vi "ZLIB Extract Stream__ogtk.vi"(4 "password (none)":string, 6 "error in (no error)":errorcluster, 7 "internal name":string, 9 "unzip Refnum":T1) -> (0 "error out":errorcluster, 2 "byte stream":string, 3 "unzip Refnum out":T1)   [LabVIEW 2014]
doc: "Extracts a file in an unzip session to a target path."
uses:
  ZLIB Unzip Handle__ogtk.ctl
panel:
  out "read only":bool
  # "Please visit http://www.OpenG.org to learn about the\nOpen Source LabVIEW software movement.\n\nNOTICE -- YOU MUST LEAVE THIS NOTICE IN PLACE.  PER THE TERMS OF THE LICENSE BELOW, YOU MAY SUBLICENSE THIS SOFTWARE \nIN ANY WAY THAT DOES NOT CONFLICT WITH THIS LICENSE.\n\n### BSD License (http://www.opensource.org/licenses/bsd-license.php) Begin ###\n \nCopyright (C) 2002-2007 Rolf Kalbermatter rolf.kalbermatter@citeng.com\nCopyright (C) 2002 Jim Kring jim@jimkring.com\n\nAll rights reserved.\n\nRedistribution and use in source and binary forms, with or without modification, are permitted provided that the following conditions are met:\n\n    * Redistributions of source code must retain the above copyright notice, this list of conditions and the following disclaimer.\n    * Redistributions in binary form must reproduce the above copyright notice, this list of conditions and the following disclaimer in the \n       documentation and/or other materials provided with the distribution.\n    * Neither the name of SciWare, James Kring, Inc., nor the names of its contributors may be used to endorse or promote products derived \n       from this software without specific prior written permission.\n\nTHIS SOFTWARE IS PROVIDED BY THE COPYRIGHT HOLDERS AND CONTRIBUTORS \"AS IS\" AND ANY EXPRESS OR IMPLIED WARRANTIES, \nINCLUDING, BUT NOT LIMITED TO, THE IMPLIED WARRANTIES OF MERCHANTABILITY AND FITNESS FOR A PARTICULAR PURPOSE ARE \nDISCLAIMED. IN NO EVENT SHALL THE COPYRIGHT OWNER OR CONTRIBUTORS BE LIABLE FOR ANY DIRECT, INDIRECT, INCIDENTAL,\n SPECIAL, EXEMPLARY, OR CONSEQUENTIAL DAMAGES (INCLUDING, BUT NOT LIMITED TO, PROCUREMENT OF SUBSTITUTE GOODS OR \nSERVICES; LOSS OF USE, DATA, OR PROFITS; OR BUSINESS INTERRUPTION) HOWEVER CAUSED AND ON ANY THEORY OF LIABILITY, \nWHETHER IN CONTRACT, STRICT LIABILITY, OR TORT (INCLUDING NEGLIGENCE OR OTHERWISE) ARISING IN ANY WAY OUT OF THE USE \nOF THIS SOFTWARE, EVEN IF ADVISED OF THE POSSIBILITY OF SUCH DAMAGE.\n\n### BSD License End ###"
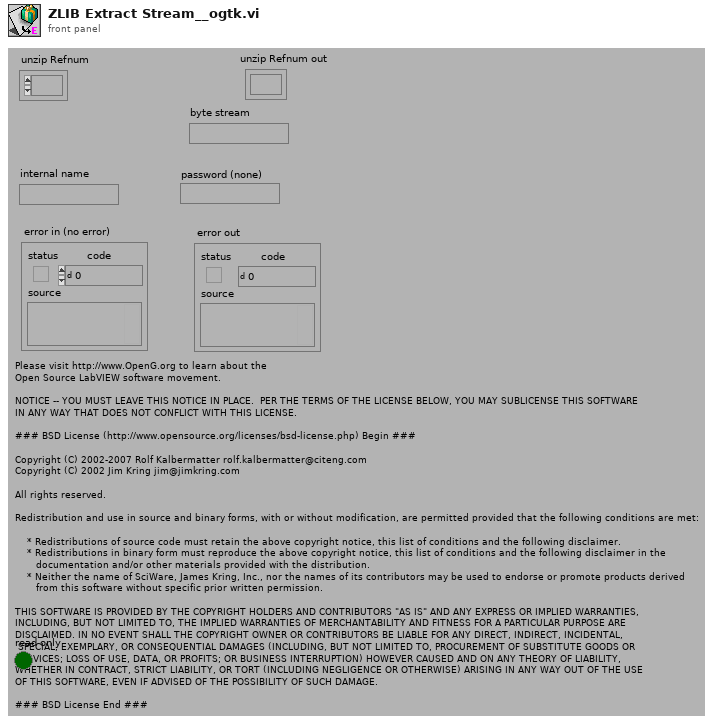
[diagram p1: front panel]
types:
  T1 = typedef "ZLIB Unzip Handle__ogtk.ctl" = refnum<k1>
  T2 = typedef "ZLIB File Info__ogtk.ctl" = cluster{"version":u32, "version needed":u32, "encrypted":bool, "flag":u32, "compression":i32, "dos date":u32, "crc":u32, "compressed size":u32, "uncompressed size":u32, "extra info":string, "file comment":string, "disk num start":u32, "internal fa":u32, "external fa":u32, "file timestamp":u32}
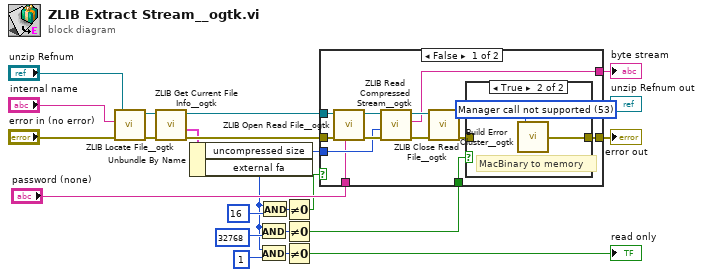
[diagram p0: block diagram]
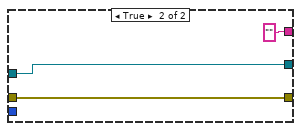
[diagram p3: hidden frame]
diagram:
  n1 = call "ZLIB Locate File__ogtk.vi"("error in (no error)"="error in (no error)", "name (empty: -)"="internal name", "unzip Refnum"="unzip Refnum") -> ("error out"=w14:errorcluster, "unzip Refnum out"=w23:T1)  [unwired: 3 in]
  n2 = call "ZLIB Get Current File Info__ogtk.vi"("error in (no error)"=w14, "unzip Refnum"=w23) -> ("error out"=w22:errorcluster, "file info"=w9:T2, "unzip Refnum out"=w17:T1)  [unwired: 6 in, 1 out]
  n3 = Unbundle By Name(w9) -> ("uncompressed size"=w20:u32, "external fa"=w5:u32)
  n4 = And(x=w5, y=u32 32768) -> (x .and. y?=w8:u32)
  n5 = And(x=w5, y=u32 1) -> (x .and. y?=w18:u32)
  n6 = And(x=w5, y=u32 16) -> (x .and. y?=w19:u32)
  n7 = Not Equal To 0?(x=w19) -> (x != 0?=w4:bool)
  n8 = Not Equal To 0?(x=w8) -> (x != 0?=w2:bool)
  n9 = Not Equal To 0?(x=w18) -> (x != 0?=→"read only":bool)
  n10 = case shown="False" w4 {
    tunnel: w22 -> [w36 w40]
    tunnel: w20 -> [w34 _]
    tunnel: w17 -> [w32 w42]
    tunnel: [w24 w40] -> w15
    tunnel: [w29 w42] -> w16
    tunnel: "password (none)" -> [w28 _]
    tunnel: [w27 "" ("byte stream")] -> w3
    tunnel: w2 -> [w26 _]
    frame False {
      n11 = call "ZLIB Open Read File__ogtk.vi"("password (none)"=w28, "error in (no error)"=w36, "unzip Refnum"=w32) -> ("error out"=w35:errorcluster, "unzip Refnum out"=w31:T1)  [unwired: 3 in, 2 out]
      n12 = call "ZLIB Read Compressed Stream__ogtk.vi"("error in (no error)"=w35, "uncompressed size"=w34, "unzip Refnum"=w31) -> ("error out"=w33:errorcluster, "byte stream"=w27:string, "unzip Refnum out"=w30:T1)  [unwired: 4 in]
      n13 = call "ZLIB Close Read File__ogtk.vi"("error in (no error)"=w33, "unzip Refnum"=w30) -> ("error out"=w25:errorcluster, "unzip Refnum out"=w29:T1)  [unwired: 8 in]
      n14 = case shown="True" w26 {
        tunnel: w25 -> [w37 _]
        tunnel: [w37 w39] -> w24
        frame False {
        }
        frame True {
          w38 = 53 items=["No error", "Argument error", "Memory is full", "Out of zone", "End of file", "File already open", "Generic file I/O error", "File not found", "File permission error", "Disk is full", "Duplicate path", "Too many files open", "System feature not enabled", "Resource file not found", "Cannot add resource", "Resource not found", "Image not found", "Image memory error", "Pen does not exist", "Config type invalid", "Config token not found", "Config parse error", "Config memory error", "Bad external code format", "Bad external code offset", "External code not present", "Null window", "Destroy window error", "Null menu", "Print aborted", "Bad print record", "Print driver error", "Windows error during printing", "Memory error during printing", "Print dialog error", "Generic print error", "Invalid device refnum", "Device not found", "Device parameter error", "Device unit error", "Cannot open device", "Device call aborted", "Generic error", "Cancelled by user", "Object ID too low", "Object ID too high", "Object not in heap", "Unknown heap", "Unknown object (invalid DefProc)", "Unknown object (DefProc not in table)", "Message out of range", "Invalid (null) method", "Unknown message", "Manager call not supported", "Bad address", "Network operation in progress", "Network operation timed out", "Connection is busy", "Network attribute not supported", "Network error", "Address in use", "System out of memory", "Connection aborted", "Connection refused", "Not connected", "Already connected", "Connection closed", "Initialization error (interapplication manager)", "Bad occurrence", "Wait on unbound occurrence handler", "Occurrence queue overflow", "Datalog type conflict", "Unused", "Unrecognized type (interapplication manager)", "Memory corrupt", "Failed to make temporary DLL", "Old CIN version", "Drag socket not found", "Failed to load drop-object", "Failed to register OLE object", "Failed to release OLE object", "Format specifier type mismatch", "Unknown format specifier", "Too few format specifiers", "Too many format specifiers", "Scan failed", "Newer CIN version", "Error converting to variant", "Runtime menu error", "Password tampered", "Variant attribute not found", "Incompatible variant data type", "Event data is not available", "Event Store is not present", "Occurrence is not found", "Event Queue is not created", "Event info is not available", "Refnum passed is NULL", "Error retrieving Class GUID", "Error retrieving CoClass GUID", "Error retrieving TypeLib GUID.", "Bad built application magic bytes.", "Specific driver is different from the specific driver associated with the Logical Name.", "There is no session opened to the class driver.", "Max Error", "MAX - Error with config objects", "MAX - Error loading configuration", "MAX - Group not supported"]
          # "MacBinary to memory"
          n15 = call "Build Error Cluster__ogtk.vi"("code"=w38) -> ("error out"=w39:errorcluster)  [unwired: 1 in]
        }
      }
    }
    frame True {
    }
  }
  "error out" <- w15
  "unzip Refnum out" <- w16
  "byte stream" <- w3
